vi "ActionVIOnCompile.vi"(8 "error in (no error)":errorcluster, 11 "Device Item Ref in":T1 format="%.0x") -> (0 "error out":errorcluster)   [LabVIEW 2020, in "FPGA Addon System Explorer.lvlib"]
uses:
  FPGA Addon System Explorer.lvlib
  <vilib>/NI VeriStand/Custom Device API/Custom Device Item Ref.ctl
  <vilib>/NI VeriStand/Custom Device API/Data Access Type.ctl
  Addon Shared/Types/FG Action.ctl
  Addon Shared/Types/Compiled.Settings.ctl
  Addon Shared/Types/Compiled.RegisterSettings.ctl
  Addon Shared/Types/Scalar Type.ctl
  Addon Shared/Types/Register Information.ctl
  Addon Shared/Types/FPGA Addon Data Type.ctl
  <vilib>/NI VeriStand/Custom Device API/Block Data Reference.ctl
  <vilib>/NI VeriStand/Custom Device API/Data Reference.ctl
  Addon Shared/Types/Compiled.DMASettings.ctl
  Addon Shared/Types/DMA Settings.ctl
  Addon Shared/Types/Delacing Scheme.ctl
  Addon Shared/Types/DMA Acquisition Mode.ctl
  <vilib>/NI VeriStand/Custom Device API/Waveform Data Reference.ctl
  Addon Shared/Types/FPGA Settings.ctl
  <vilib>/NI VeriStand/Custom Device API/Custom Device Target Type.ctl
  Addon Shared/SubVIs/Constants.vi
  <vilib>/NI VeriStand/Custom Device API/NI VeriStand - Get Item Property.vi
  <vilib>/NI VeriStand/Custom Device API/Get Item Property (Path).vi
  <vilib>/NI VeriStand/Custom Device API/Get Item Property (String).vi
  <vilib>/NI VeriStand/Custom Device API/Get Item Property (Boolean).vi
  <vilib>/NI VeriStand/Custom Device API/Set Item Property (Path).vi
  <vilib>/NI VeriStand/Custom Device API/Set Item Property (String).vi
  <vilib>/NI VeriStand/Custom Device API/Set Item Property (Boolean).vi
  <vilib>/NI VeriStand/Custom Device Tools/Custom Device Utility Library/NI VeriStand - Search for Item.vi
  <vilib>/NI VeriStand/Custom Device Tools/Custom Device Utility Library/NI VeriStand - Search for Item by GUID.vi
  SubVIs/Get Scalar Datatypes and Refs.vi
  <vilib>/NI VeriStand/Custom Device API/Set Item Property (Variant).vi
  <vilib>/NI VeriStand/Custom Device API/Custom Device API.lvlib
  Addon Shared/FPGA Addon Shared.lvlib
  <vilib>/NI/NIVS Inline Async API/_Data Access System Explorer/Data Access System Explorer.lvlib
  <vilib>/NI VeriStand/Custom Device Tools/Custom Device Utility Library/Custom Device Utility Library.lvlib
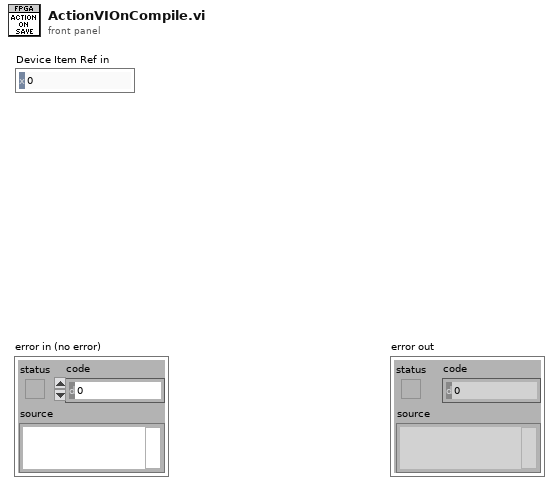
[diagram p1: front panel]
types:
  T1 = typedef "Custom Device API.lvlib/Custom Device Item Ref.ctl" = u64
  T2 = typedef "FPGA Addon Shared.lvlib/Compiled.Settings.ctl" = cluster{"Name":string, "IncomingRegisters.Settings":T3[], "IncomingRegisters.Refs":cluster{"Refs":T7[], "Values":dbl[]}, "OutgoingRegisters.Settings":T3[], "OutgoingRegisters.Refs":cluster{"Refs":T7[], "Values":dbl[]}, "Incoming.Size":i32, "Outgoing.Size":i32, "IncomingDMA.Settings":T9[], "OutgoingDMA.Settings":T9[], "FPGA.Settings":T14, "Target.Type":T15}
  T3 = typedef "FPGA Addon Shared.lvlib/Compiled.RegisterSettings.ctl" = cluster{"Scalar Type":T4, "Index":i32, "Length":i32, "Register":T5}
  T4 = typedef "FPGA Addon Shared.lvlib/Scalar Type.ctl" = enum16{"Standard", "Bitpacked"}
  T5 = typedef "FPGA Addon Shared.lvlib/Register Information.ctl" = cluster{"Name":string, "Data Type":T6, "Default Value":variant, "Attributes":variant}
  T6 = typedef "FPGA Addon Shared.lvlib/FPGA Addon Data Type.ctl" = enum8{"<Null>", "I8", "I16", "I32", "I64", "U8", "U16", "U32", "U64", "SGL", "Boolean", "Analog PWM In Settings", "Analog PWM In", "Digital PWM In Settings", "Digital PWM In", "Digital PWM Out", "Sine Out", "FXP", "FXP+/-24.5", "FXP+/-16.5", "FXP+/-32.8", "FXP+/-64.32", "FXP+/-16.7", "FXP+/-20.5", "FXP+/-27.5", "FXP+/-32.16", "FXP+16.3", "FXP+18.3", "Digital Static In", "Digital Static Out", "Digital Static In Settings", "Digital WSS Out", "Quad Encoder Settings", "Quad Encoder In", "Group"}
  T7 = typedef "Custom Device API.lvlib/Block Data Reference.ctl" = cluster{"Data Reference":T8, "Offset":u64, "Length":u64}
  T8 = typedef "Custom Device API.lvlib/Data Reference.ctl" = i32
  T9 = typedef "FPGA Addon Shared.lvlib/Compiled.DMASettings.ctl" = cluster{"Name":string, "Data Type":T6, "DMA.Settings":T10, "DMA.VSRefs":T13[]}
  T10 = typedef "FPGA Addon Shared.lvlib/DMA Settings.ctl" = cluster{"Number of Channels":u8, "Delacing Scheme":T11, "Update Rate":u32, "dt":dbl, "Mode":T12, "Number of Samples":u32, "DMA Host Buffer":u32}
  T11 = typedef "FPGA Addon Shared.lvlib/Delacing Scheme.ctl" = enum8{"Interleaved", "Bitpacked"}
  T12 = typedef "FPGA Addon Shared.lvlib/DMA Acquisition Mode.ctl" = enum8{"Continuous", "Triggered Finite"}
  T13 = typedef "Custom Device API.lvlib/Waveform Data Reference.ctl" = i32
  T14 = typedef "FPGA Addon Shared.lvlib/FPGA Settings.ctl" = cluster{"Bitfile path":path, "RIO Device Address":string, "Group":bool}
  T15 = typedef "Custom Device API.lvlib/Custom Device Target Type.ctl" = enum16{"PharLap", "VxWorks", "Windows", "Linux_32_ARM", "Linux_x64"}
  T16 = typedef "Custom Device API.lvlib/Data Access Type.ctl" = enum16{"Read", "Write"}
  T17 = typedef "FPGA Addon Shared.lvlib/FG Action.ctl" = enum8{"GET", "SET"}
  T18 = typedef "Custom Device API.lvlib/Custom Device Item Info.ctl" = cluster{"Name":string, "Is Channel":bool, "GUID":string, "Is Waveform":bool}
  T19 = cluster{"Name":string, "Type":enum16{"Output/Write", "Input/Read", "Input/ReadWrite"}, "VS Refs":T1[]}[]
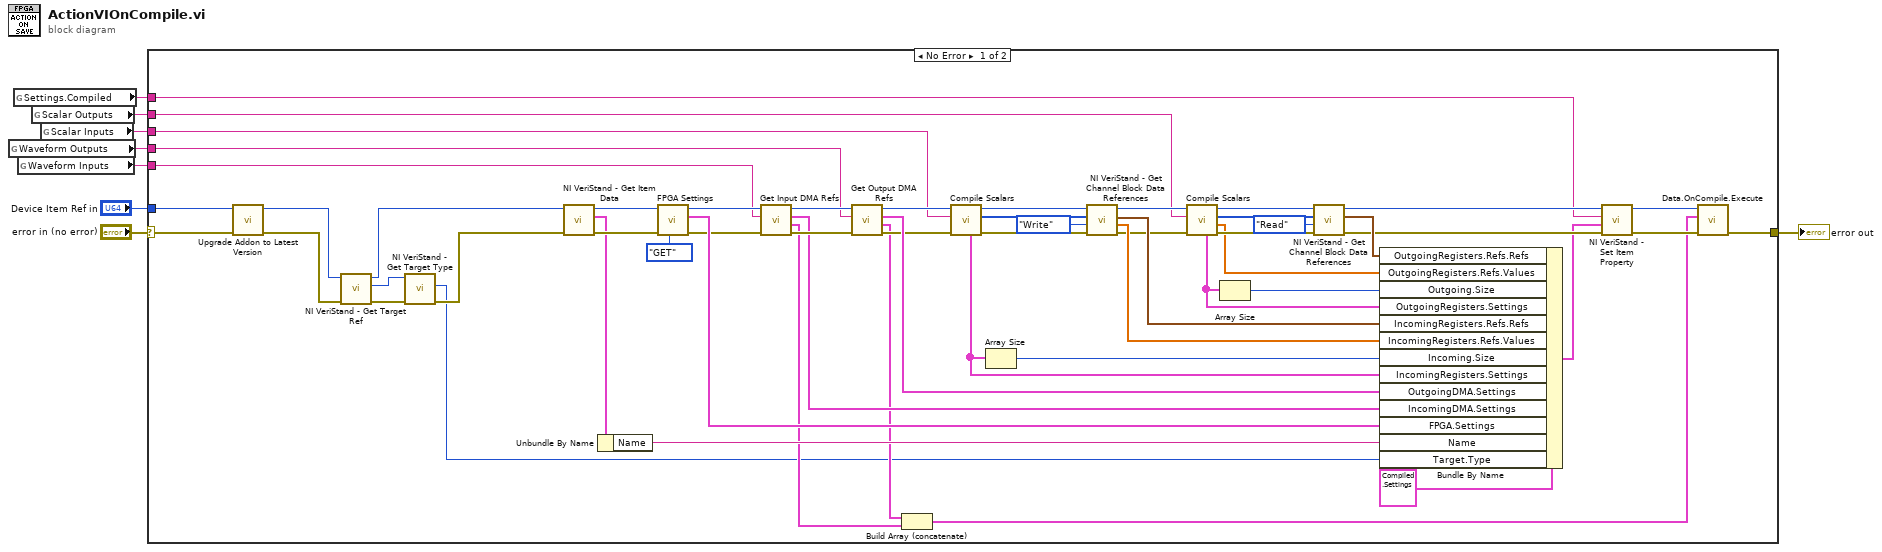
[diagram p0: block diagram]
diagram:
  n1 = global read "Constants.vi" "Waveform Outputs"() -> (w4:string)
  n2 = global read "Constants.vi" "Settings.Compiled"() -> (w1:string)
  n3 = global read "Constants.vi" "Waveform Inputs"() -> (w5:string)
  n4 = global read "Constants.vi" "Scalar Outputs"() -> (w2:string)
  n5 = global read "Constants.vi" "Scalar Inputs"() -> (w3:string)
  n6 = case shown="No Error" "error in (no error)" {
    selector: "error in (no error)" -> [w12 w65]
    tunnel: [w21 w65] -> w7
    tunnel: "Device Item Ref in" -> [w11 _]
    tunnel: w5 -> [w31 _]
    tunnel: w4 -> [w30 _]
    tunnel: w3 -> [w29 _]
    tunnel: w2 -> [w28 _]
    tunnel: w1 -> [w25 _]
    frame No Error {
      n7 = call "Upgrade Addon to Latest Version.vi"("error in (no error)"=w12, "Device Item Ref in in"=w11) -> ("error out"=w10:errorcluster, "Device Item Ref out"=w9:T1)  [unwired: 8 in]
      n8 = call <vilib>:"NI VeriStand - Get Target Ref.vi"("error in"=w10, "Item Ref in"=w9) -> ("error out"=w18:errorcluster, "Target Ref"=w17:T1, "Item Ref out"=w15:T1)  [unwired: 6 in, 1 out]
      n9 = call <vilib>:"NI VeriStand - Get Target Type.vi"("error in (no error)"=w18, "Item Ref in"=w17) -> ("error out"=w16:errorcluster, "Target Type"=w14:T15)  [unwired: 7 in, 1 out]
      n10 = call <vilib>:"NI VeriStand - Get Item Data.vi"("error in (no error)"=w16, "Item Ref in"=w15) -> ("error out"=w62:errorcluster, "Item Info"=w50:T18, "Item Ref out"=w61:T1)  [unwired: 6 in, 1 out]
      n11 = Unbundle By Name(w50) -> ("Name"=w51:string)
      n12 = call "FPGA Settings.vi"("Action"=FG_Action."GET", "error in (no error)"=w62, "Item Ref"=w61) -> ("error out"=w63:errorcluster, "FPGA Settings"=w64:T14, "Item Ref out"=w52:T1)  [unwired: 6 in]
      n13 = call "Get Input DMA Refs.vi"("error in (no error)"=w63, "Item GUID"=w31, "Section Ref in"=w52) -> ("error out"=w54:errorcluster, "Refs"=w24:T19, "DMA Settings"=w53:T9[], "Section Ref out"=w56:T1)  [unwired: 5 in]
      n14 = call "Get Output DMA Refs.vi"("error in (no error)"=w54, "Item GUID"=w30, "Section Ref in"=w56) -> ("error out"=w55:errorcluster, "Refs"=w23:T19, "DMA"=w58:T9[], "Section Ref out"=w57:T1)  [unwired: 5 in]
      n15 = Build Array (concatenate)(w23, w24) -> (w19:T19)
      n16 = call "Compile Scalars.vi"("error in (no error)"=w55, "Item GUID"=w29, "Section Ref in"=w57) -> ("error out"=w36:errorcluster, "VS Ref"=w34:T1[], "Section Ref out"=w35:T1, "Registers Ref"=w59:T3[])  [unwired: 4 in, 1 out]
      n17 = Array Size(array=w59) -> (size(s)=w48:i32)
      n18 = call <vilib>:"NI VeriStand - Get Channel Block Data References.vi"("error in (no error)"=w36, "Access"=Data_Access_Type."Write", "Channel Refs"=w34, "Device Ref in"=w35) -> ("error out"=w37:errorcluster, "Values Array"=w49:dbl[], "Block Data Refs"=w45:T7[], "Device Ref out"=w38:T1)  [unwired: 4 in]
      n19 = call "Compile Scalars.vi"("error in (no error)"=w37, "Item GUID"=w28, "Section Ref in"=w38) -> ("error out"=w40:errorcluster, "Default Values"=w13:dbl[], "VS Ref"=w42:T1[], "Section Ref out"=w41:T1, "Registers Ref"=w60:T3[])  [unwired: 4 in]
      n20 = Array Size(array=w60) -> (size(s)=w47:i32)
      n21 = call <vilib>:"NI VeriStand - Get Channel Block Data References.vi"("error in (no error)"=w40, "Access"=Data_Access_Type."Read", "Channel Refs"=w42, "Device Ref in"=w41) -> ("error out"=w32:errorcluster, "Block Data Refs"=w46:T7[], "Device Ref out"=w26:T1)  [unwired: 4 in, 1 out]
      n22 = Bundle By Name(cluster=T2 {"Name"="", "IncomingRegisters.Settings"=[], "IncomingRegisters.Refs"={"Refs"=[], "Values"=[]}, "OutgoingRegisters.Settings"=[], "OutgoingRegisters.Refs"={"Refs"=[], "Values"=[]}, "Incoming.Size"=0, "Outgoing.Size"=0, "IncomingDMA.Settings"=[], "OutgoingDMA.Settings"=[], "FPGA.Settings"={"Bitfile path"=path "", "RIO Device Address"="", "Group"=FALSE}, "Target.Type"=enum."PharLap"}, "OutgoingRegisters.Refs.Refs"=w46, "OutgoingRegisters.Refs.Values"=w13, "Outgoing.Size"=w47, "OutgoingRegisters.Settings"=w60, "IncomingRegisters.Refs.Refs"=w45, "IncomingRegisters.Refs.Values"=w49, "Incoming.Size"=w48, "IncomingRegisters.Settings"=w59, "OutgoingDMA.Settings"=w58, "IncomingDMA.Settings"=w53, "FPGA.Settings"=w64, "Name"=w51, "Target.Type"=w14) -> (w27:T2)
      n23 = call-poly <vilib>:"NI VeriStand - Set Item Property.vi"("error in (no error)"=w32, "Value"=w27, "Property Name"=w25, "Item Ref in"=w26) -> ("error out"=w22:errorcluster, "Item Ref out"=w20:T1)  [unwired: 5 in, 1 out]
      n24 = call <vilib>:"Data.OnCompile.Execute.vi"("error in"=w22, "VS Ref Groups"=w19, "Custom Device Ref"=w20) -> ("error out"=w21:errorcluster)  [unwired: 7 in, 1 out]
    }
    frame Error {
    }
  }
  "error out" <- w7
